vi "Stop.vi"(8 "error in (no error)":errorcluster, 10 "Parameters":dbl[](array[numeric]), 11 "SoftmotionAxis in":refnum<class "SoftmotionAxis.lvclass">) -> (0 "error out":errorcluster, 3 "SoftmotionAxis out":refnum<class "SoftmotionAxis.lvclass">)   [LabVIEW 2017, in "SoftmotionAxis.lvclass"]
uses:
  SoftmotionAxis.lvclass
  <resource>/objmgr/nimotion.rc
  Utilities/WordManipulationLibrary.lvlib
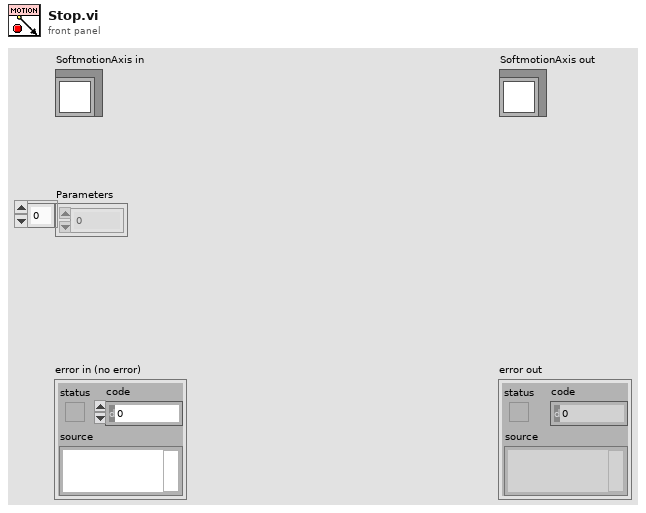
[diagram p1: front panel]
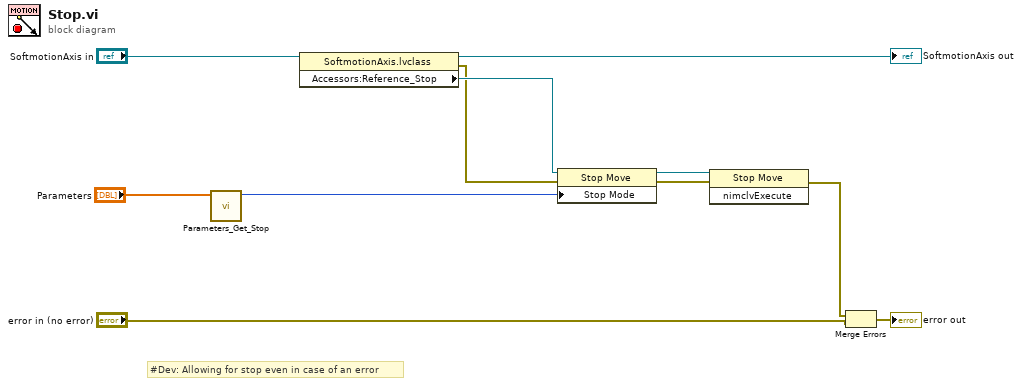
[diagram p0: block diagram]
diagram:
  # "#Dev: Allowing for stop even in case of an error"
  n1 = call "Parameters_Get_Stop.vi"("Parameters"="Parameters") -> ("Stop Mode"=w5:i32)  [unwired: 10 in]
  n2 = property class="SoftmotionAxis.lvclass"(reference="SoftmotionAxis in") -> (reference out=→"SoftmotionAxis out":refnum<class "SoftmotionAxis.lvclass">, error out=w7:errorcluster, "Accessors:Reference_Stop"=w8:refnum<k20>)  [unwired: 1 in]
  n3 = property class="Stop Move"(reference=w8, error in=w7, "Stop Mode"=w5) -> (reference out=w1:refnum<k20>, error out=w6:errorcluster)
  n4 = invoke class="Stop Move" method="nimclvExecute"(reference=w1, error in=w6) -> (error out=w3:errorcluster)  [unwired: 1 in, 2 out]
  n5 = Merge Errors(w3, "error in (no error)") -> (→"error out":errorcluster)
